vi "Update Status.vi"() -> ()   [LabVIEW 2021, in "Class 1.lvclass"]
uses:
  Class 1/Class 1.lvclass
  C:/Users/enProducts/Downloads/KIA_Enproducts/KIA_Enproducts/User Interface/Main Panel/Test Screen/Controls/Test Screen UE MSG.ctl
  C:/Users/enProducts/Downloads/KIA_Enproducts/KIA_Enproducts/User Interface/Main Panel/Test Screen/Controls/Test Screen UE CMD.ctl
panel:
  out "Cluster":cluster{"Cluster":cluster{"Part ID":string}}
  out "Serial Number":dbl
  in  "error in":errorcluster
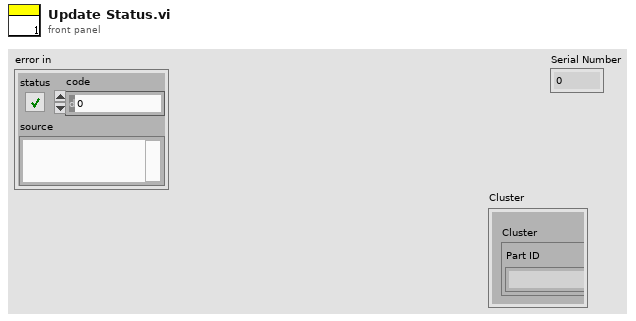
[diagram p1: front panel]
types:
  T1 = typedef "Test Screen UE MSG.ctl" = cluster{"TS UE CMDs":T2, "Data":variant}
  T2 = typedef "Test Screen UE CMD.ctl" = enum16{"Update Model", "Update Expected Barcode", "Status Update", "Error Popup", "Update Scanned Barcode Field", "Test Running Status", "Test Result Update", "Update Torque Results", "Reprint Pop Up Open", "Reprint pop up close", "Communication Status Update", "Rescan Reprint Pop Open", "Rescan Reprint Pop Close"}
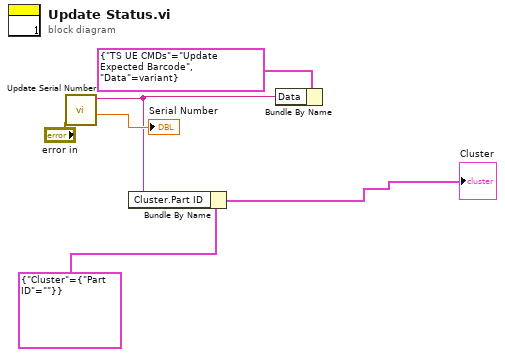
[diagram p0: block diagram]
diagram:
  n1 = call "Update Serial Number.vi"("error in"="error in") -> ("Serial Number"=→"Serial Number":dbl, "Serial number"=w3:string)  [unwired: 8 in, 1 out]
  n2 = Bundle By Name(cluster=cluster{"Cluster":cluster{"Part ID":string}} {"Cluster"={"Part ID"=""}}, "Cluster.Part ID"=w3) -> (→"Cluster":cluster{"Cluster":cluster{"Part ID":string}})
  n3 = Bundle By Name(cluster=T1 {"TS UE CMDs"=enum."Update Expected Barcode", "Data"=variant} ("TS UE CMD"), "Data"=w3) -> ()  [unwired: 1 out]
